vi "Reset Transform.vi"(8 "error in (no error)":errorcluster, 11 "Canvas in":refnum<class "Drawer .Net.lvclass">) -> (0 "error out":errorcluster, 3 "Canvas out":refnum<class "Drawer .Net.lvclass">)   [LabVIEW 2023, in "Glyph .NET.lvlib" / "Drawer .Net.lvclass"]
uses:
  Drawer .Net.lvclass
  Drawer .Net.lvclass/Drawer .Net.ctl
  Read Graphics.vi
  System.Drawing
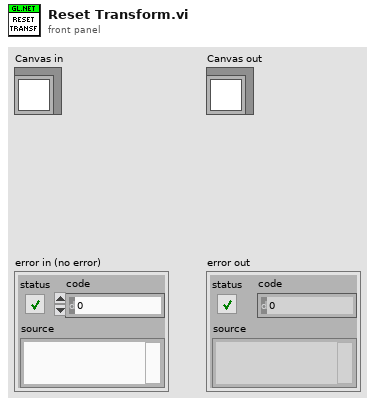
[diagram p1: front panel]
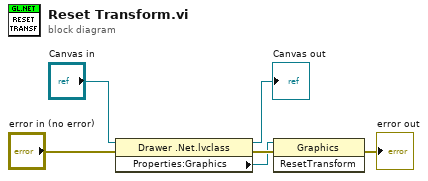
[diagram p0: block diagram]
diagram:
  n1 = property class="Drawer .Net.lvclass"(reference="Canvas in", error in="error in (no error)") -> (reference out=→"Canvas out":refnum<class "Drawer .Net.lvclass">, error out=w5:errorcluster, "Properties:Graphics"=w3:refnum<k24>)
  n2 = invoke class="Graphics" method="ResetTransform"(reference=w3, error in=w5) -> (error out=→"error out":errorcluster)  [unwired: 1 in, 2 out]
